vi "Create Metadata Response.vi"(8 "error in (no error)":errorcluster, 9 "gRPCid":T9, 10 "MeasurementPluginService in":refnum<class "Measurement Plugin Service.lvclass">) -> (0 "error out":errorcluster, 2 "Get Metadata Response":T1, 3 "gRPCid out":T9)   [LabVIEW 2020, in "MeasurementLink Measurement Server.lvlib" / "IMeasurement Service.lvclass"]
uses:
  IMeasurement Service.lvclass
  <vilib>/gRPC/LabVIEW gRPC Library/Shared/grpcId.ctl
  Helpers/TypeDefs/GetMetadataResponse.ctl
  Helpers/TypeDefs/Measurement Details.ctl
  Helpers/TypeDefs/MeasurementSignature.ctl
  Helpers/TypeDefs/ConfigurationParameter.ctl
  Helpers/TypeDefs/Parameter_AnnotationsEntry.ctl
  <vilib>/gRPC/LabVIEW gRPC Library/Shared/Any.ctl
  Helpers/TypeDefs/OutputParameter.ctl
  Helpers/TypeDefs/UserInterfaceDetails.ctl
  Measurement Plugin Service/Measurement Plugin Service.lvclass
  <vilib>/gRPC/LabVIEW gRPC Library/Server API/typeDefs/gRPC Status Code.ctl
  MeasurementLink Measurement Server.lvlib
  <vilib>/gRPC/LabVIEW gRPC Library/grpc-lvsupport-release.lvlib
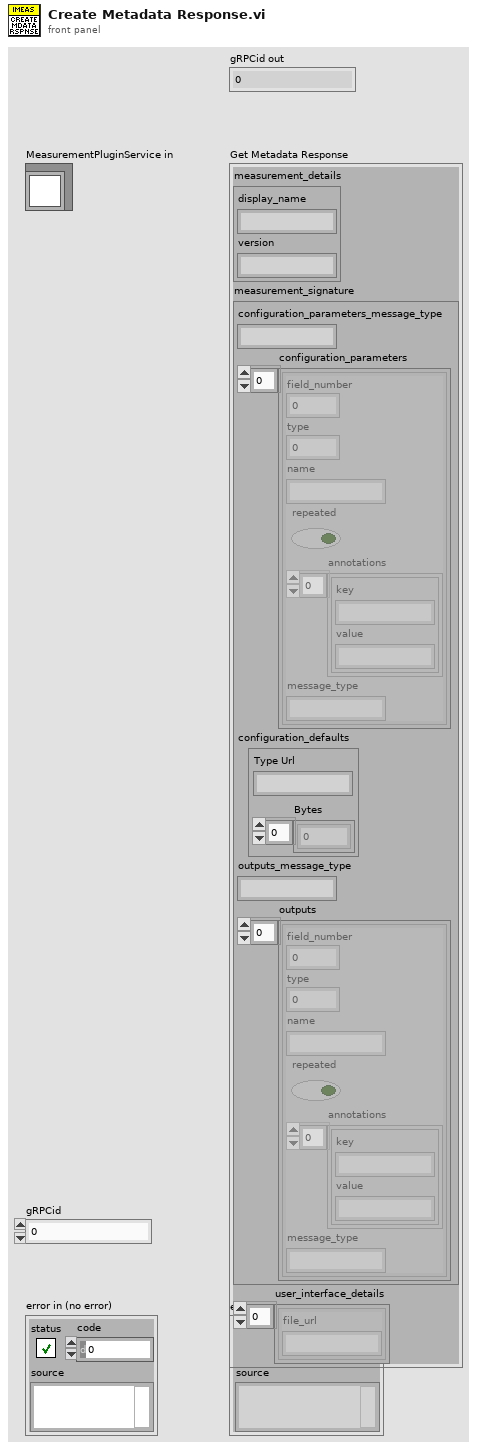
[diagram p1: front panel]
types:
  T1 = typedef "MeasurementLink Measurement Server.lvlib/GetMetadataResponse.ctl" = cluster{"measurement_details":T2, "measurement_signature":T3, "user_interface_details":T8[]}
  T2 = typedef "MeasurementLink Measurement Server.lvlib/Measurement Details.ctl" = cluster{"display_name":string, "version":string}
  T3 = typedef "MeasurementLink Measurement Server.lvlib/MeasurementSignature.ctl" = cluster{"configuration_parameters_message_type":string, "configuration_parameters":T4[], "configuration_defaults":T6, "outputs_message_type":string, "outputs":T7[]}
  T4 = typedef "MeasurementLink Measurement Server.lvlib/ConfigurationParameter.ctl" = cluster{"field_number":i32, "type":i32, "name":string, "repeated":bool, "annotations":T5[], "message_type":string}
  T5 = typedef "MeasurementLink Measurement Server.lvlib/Parameter_AnnotationsEntry.ctl" = cluster{"key":string, "value":string}
  T6 = typedef "grpc-lvsupport-release.lvlib/Any.ctl" = cluster{"Type Url":string, "Bytes":u8[]}
  T7 = typedef "MeasurementLink Measurement Server.lvlib/OutputParameter.ctl" = cluster{"field_number":i32, "type":i32, "name":string, "repeated":bool, "annotations":T5[], "message_type":string}
  T8 = typedef "MeasurementLink Measurement Server.lvlib/UserInterfaceDetails.ctl" = cluster{"file_url":string}
  T9 = typedef "grpc-lvsupport-release.lvlib/grpcId.ctl" = u64
  T10 = typedef "grpc-lvsupport-release.lvlib/gRPC Status Code.ctl" = enum16{"OK", "CANCELLED", "UNKNOWN", "INVALID_ARGUMENT", "DEADLINE_EXCEEDED", "NOT_FOUND", "ALREADY_EXISTS", "PERMISSION_DENIED", "RESOURCE_EXHAUSTED", "FAILED_PRECONDITION", "ABORTED", "OUT_OF_RANGE", "UNIMPLEMENTED", "INTERNAL", "UNAVAILABLE", "DATA_LOSS", "UNAUTHENTICATED"}
  T11 = typedef "MeasurementLink Measurement Server.lvlib/Measurement Plugin Service.lvclass/Plugin Paths.ctl" = cluster{"Get Measurement Details VI Path":path, "Get Type Specializations VI Path":path, "Get UI Details VI Path":path, "Measurement Logic VI Path":path, "Measurement Configuration CTL Path":path, "Measurement Results CTL Path":path}
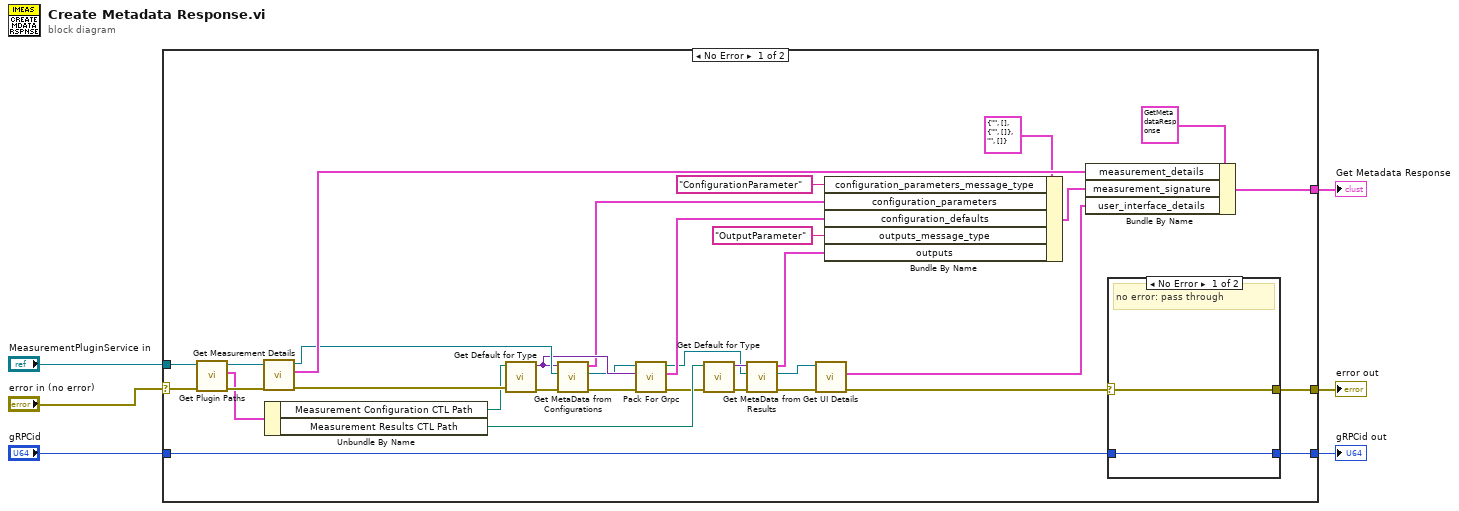
[diagram p0: block diagram]
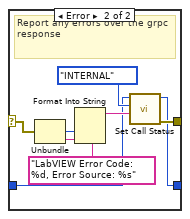
[diagram p2: hidden frame]
diagram:
  n1 = case shown="No Error" "error in (no error)" {
    selector: "error in (no error)" -> [w10 w53]
    tunnel: [w35 w52] -> w6
    tunnel: "gRPCid" -> [w34 w52]
    tunnel: [w33 w53] -> w4
    tunnel: [w31 _] -> w3
    tunnel: "MeasurementPluginService in" -> [w27 _]
    frame No Error {
      n2 = call-dynamic "Get Plugin Paths.vi"("error in (no error)"=w10, "MeasurementPluginService in"=w27) -> ("error out"=w38:errorcluster, "Plugin Paths"=w28:T11, "MeasurementPluginService out"=w36:refnum<class "Measurement Plugin Service.lvclass">)  [unwired: 7 in]
      n3 = call-dynamic "Get Measurement Details.vi"("error in"=w38, "MeasurementPluginService in"=w36) -> ("error out"=w39:errorcluster, "Measurement Details"=w40:T2, "MeasurementPluginService out"=w37:refnum<class "Measurement Plugin Service.lvclass">)  [unwired: 5 in, 2 out]
      n4 = Unbundle By Name(w28) -> ("Measurement Configuration CTL Path"=w29:path, "Measurement Results CTL Path"=w30:path)
      n5 = call "Get Default for Type.vi"("error in (no error)"=w39, "Path of Type"=w29) -> ("error out"=w16:errorcluster, "Default for Type"=w23:variant)  [unwired: 8 in]
      n6 = call "Get MetaData from Configurations.vi"("error in"=w16, "measurement plugin service in"=w37, "configuration cluster"=w23) -> ("error out"=w22:errorcluster, "measurement plugin service out"=w8:refnum<class "Measurement Plugin Service.lvclass">, "configuration_parameters"=w11:T4[])  [unwired: 6 in]
      n7 = call-dynamic "Pack For Grpc.vi"("error in (no error)"=w22, "Data Value"=w23, "MeasurementPluginService in"=w8) -> ("error out"=w25:errorcluster, "Any"=w24:T6, "MeasurementPluginService out"=w9:refnum<class "Measurement Plugin Service.lvclass">)  [unwired: 6 in]
      n8 = call "Get Default for Type.vi"("error in (no error)"=w25, "Path of Type"=w30) -> ("error out"=w21:errorcluster, "Default for Type"=w20:variant)  [unwired: 8 in]
      n9 = call "Get MetaData from Results.vi"("error in"=w21, "measurement plugin service in"=w9, "results cluster"=w20) -> ("error out"=w15:errorcluster, "measurement plugin service out"=w7:refnum<class "Measurement Plugin Service.lvclass">, "outputs"=w12:T7[])  [unwired: 6 in]
      n10 = call-dynamic "Get UI Details.vi"("error in"=w15, "MeasurementPluginService in"=w7) -> ("error out"=w32:errorcluster, "user_interface_details"=w26:T8[])  [unwired: 7 in, 1 out]
      n11 = Bundle By Name(cluster=T3 {"configuration_parameters_message_type"="", "configuration_parameters"=[], "configuration_defaults"={"Type Url"="", "Bytes"=[]}, "outputs_message_type"="", "outputs"=[]} ("ni_measurements_v1_MeasurementSignature"), "configuration_parameters_message_type"="ConfigurationParameter" ("configuration_parameters_messagetype"), "configuration_parameters"=w11, "configuration_defaults"=w24, "outputs_message_type"="OutputParameter" ("configuration_parameters_messagetype"), "outputs"=w12) -> (w18:T3)
      n12 = Bundle By Name(cluster=T1 {"measurement_details"={"display_name"="", "version"=""}, "measurement_signature"={"configuration_parameters_message_type"="", "configuration_parameters"=[], "configuration_defaults"={"Type Url"="", "Bytes"=[]}, "outputs_message_type"="", "outputs"=[]}, "user_interface_details"=[]} ("package_templatemessage"), "measurement_details"=w40, "measurement_signature"=w18, "user_interface_details"=w26) -> (w31:T1)
      n13 = case shown="No Error" w32 {
        selector: w32 -> [w41 w45]
        tunnel: [w41 w46] -> w33
        tunnel: w34 -> [w42 w44]
        tunnel: [w42 w43] -> w35
        frame No Error {
          # "no error: pass through"
        }
        frame Error {
          # "Report any errors over the grpc response"
          n14 = Unbundle(w45) -> ("code"=w49:i32, "source"=w50:string)  [unwired: 1 out]
          n15 = Format Into String(format string="LabVIEW Error Code: %d, Error Source: %s", w49, w50) -> (resulting string=w51:string)  [unwired: 2 in, 1 out]
          n16 = call <vilib>:"Set Call Status.vi"("Details"=w51, "Status Code"=gRPC_Status_Code."INTERNAL", "gRPCid in"=w44) -> ("error out"=w46:errorcluster, "gRPCid out"=w43:T9)  [unwired: 7 in]
        }
      }
    }
    frame Error {
    }
  }
  "gRPCid out" <- w6
  "error out" <- w4
  "Get Metadata Response" <- w3
